vi "Boolean2String.vi"(11 "Boolean":bool) -> (3 "string":string)   [LabVIEW 2013]
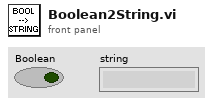
[diagram p1: front panel]
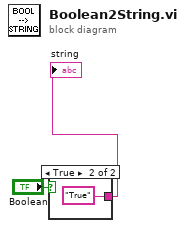
[diagram p0: block diagram]
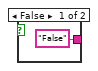
[diagram p2: hidden frame]
diagram:
  n1 = case shown="True" "Boolean" {
    tunnel: ["False" ("string") "True" ("string")] -> w2
    frame False {
    }
    frame True {
    }
  }
  "string" <- w2
